vi "ProdaNG.Tree.Selection.GetAll.vi"(7 "TestStepsTree":refnum<vi>, 8 "error in (no error)":errorcluster) -> (0 "error out":errorcluster, 1 "Selected elements values":T1[](array[typedef]), 2 "Selected elements":T2[](array[typedef]))   [LabVIEW 2016]
uses:
  ProdaNG.Tree.Fglb.Data.ctl
  ProdaNG.Tree.Fglb.Element.ctl
  ProdaNG.Tree.Fglb.Value.ctl
  ProdaNG.Tree.Fglb.Action.ctl
  ProdaNG.Configurator.Glb.vi
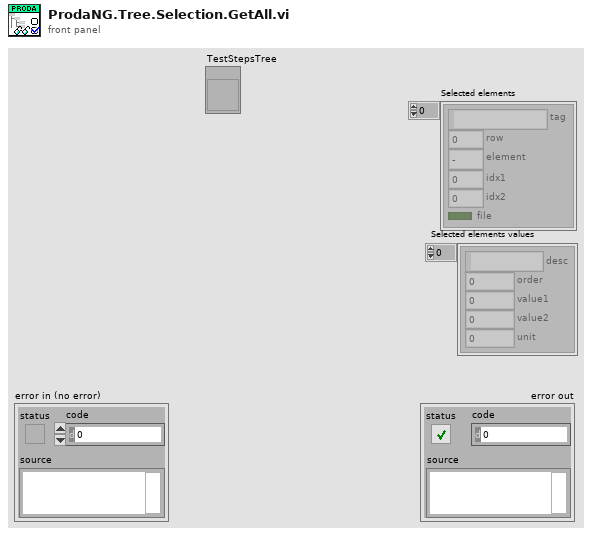
[diagram p1: front panel]
types:
  T1 = typedef "ProdaNG.Tree.Fglb.Value.ctl" = cluster{"desc":string, "order":i32, "value1":dbl, "value2":dbl, "unit":i32}
  T2 = typedef "ProdaNG.Tree.Fglb.Data.ctl" = cluster{"tag":string, "row":i32, "element":T3, "idx1":i32, "idx2":i32, "file":bool}
  T3 = typedef "ProdaNG.Tree.Fglb.Element.ctl" = enum16{"-", "PP", "TS", "TP", "TV"}
  T4 = typedef "ProdaNG.Tree.Fglb.Action.ctl" = enum16{"init", "add", "get by row", "get by tag", "get by idx"}
  T5 = typedef "ProdaNG.ProcessStepParam.ctl" = cluster{"i_id":i32, "processStepId":i32, "unitId":i32, "contentId":string, "previewId":string, "value":dbl, "valueText":string, "paramSequence":i32, "history":i32, "mdReason":string, "mdUser":string, "mdTime":string, "description":string}
  T6 = cluster{"description":string, "paramSequence":i32, "value":dbl, dbl, "unitId":i32}
  T7 = typedef "ProdaNG.TestStep.ctl" = cluster{"i_id":i32, "processStepId":i32, "testSequence":i32, "testOrder":i32, "mdReason":string, "mdUser":string, "mdTime":string, "description":string}
  T8 = typedef "ProdaNG.TestStepParam.ctl" = cluster{"i_id":i32, "testStepId":i32, "unitId":i32, "contentId":string, "previewId":string, "value":dbl, "valueText":string, "paramSequence":i32, "history":i32, "mdReason":string, "mdUser":string, "mdTime":string, "description":string}
  T9 = typedef "ProdaNG.TestValue.ctl" = cluster{"i_id":i32, "testStepId":i32, "releaseId":i32, "unitId":i32, "contentId":string, "previewId":string, "maximum":dbl, "minimum":dbl, "valueText":string, "testValueSequence":i32, "history":i32, "mdReason":string, "mdUser":string, "mdTime":string, "description":string}
  T10 = cluster{"description":string, "testSequence":i32, dbl, dbl, "unitId":i32}
  T11 = cluster{"description":string, "testValueSequence":i32, "minimum":dbl, "maximum":dbl, "unitId":i32}
  T12 = cluster{"element":T3, "found entry":T2, cluster{"description":string, "testValueSequence":i32, "minimum":dbl, "maximum":dbl, "unitId":i32}}
  T13 = cluster{"element":T3, "found entry":T2, cluster{"description":string, "testValueSequence":i32, "minimum":dbl, "maximum":dbl, "unitId":i32}}[]
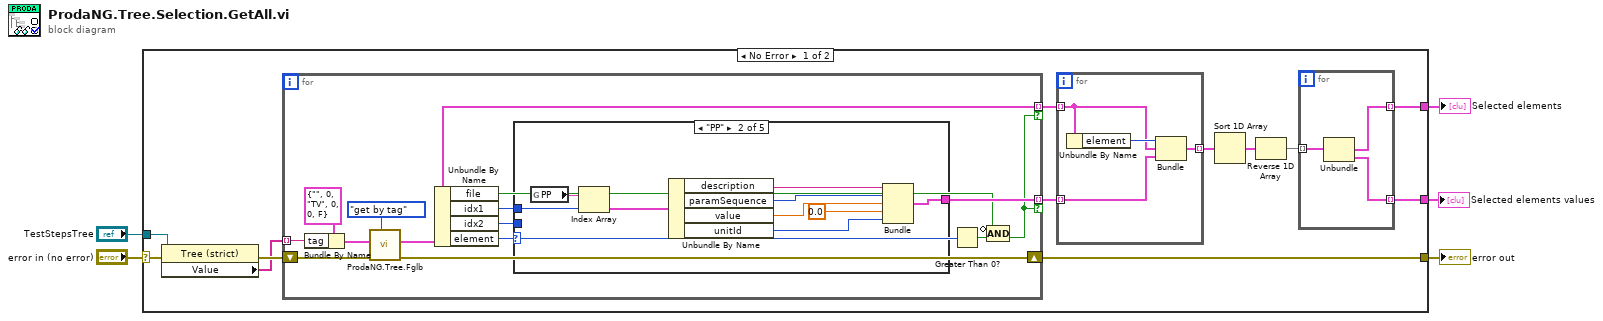
[diagram p0: block diagram]
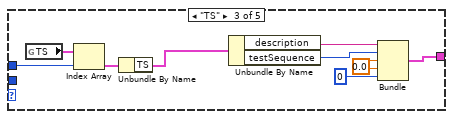
[diagram p3: hidden frame]
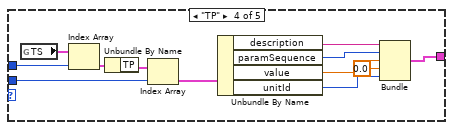
[diagram p4: hidden frame]
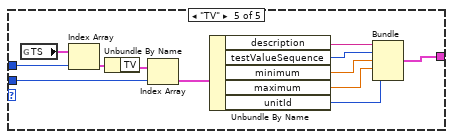
[diagram p5: hidden frame]
diagram:
  n1 = case shown="No Error" "error in (no error)" {
    selector: "error in (no error)" -> [w17 w81]
    tunnel: "TestStepsTree" -> [w14 _]
    tunnel: [w15 w81] -> w5
    tunnel: [w8 _] -> w2
    tunnel: [w6 _] -> w1
    frame No Error {
      n2 = property on="Property Node" class="Tree (strict)"(reference=w14, error in=w17) -> (error out=w16:errorcluster, "Value"=w13:string[])  [unwired: 1 out]
      n3 = for {
        tunnel: w13 -> [w35] mode=indexing
        shift-right: [w32] -> w15
        shift-left: w16 -> [w34]
        tunnel: [w33] -> w9 mode=indexing if=w26
        tunnel: [w29] -> w7 mode=indexing if=w26
        n4 = Bundle By Name(cluster=T2 {"tag"="", "row"=0, "element"=enum."TV", "idx1"=0, "idx2"=0, "file"=FALSE} ("entry in"), "tag"=w35) -> (w36:T2)
        n5 = call "ProdaNG.Tree.Fglb.vi"("Action (add)"=ProdaNG.Tree.Fglb.Action."get by tag", "error in"=w34, "entry in"=w36) -> ("error out"=w32:errorcluster, "found entry"=w33:T2)  [unwired: 6 in, 1 out]
        n6 = Unbundle By Name(w33) -> ("file"=w25:bool, "idx1"=w30:i32, "idx2"=w31:i32, "element"=w28:T3)
        n7 = case shown="\"PP\"" w28 {
          tunnel: w31 -> [_ _ _ w65 w77]
          tunnel: w30 -> [_ w44 w53 w64 w76]
          tunnel: [_ w42 w50 w60 w72] -> w29
          frame "-" {
          }
          frame "PP" {
            n8 = global read "ProdaNG.Configurator.Glb.vi" "PP"() -> (w47:T5[])
            n9 = Index Array(array=w47, index=w44) -> (element=w43:T5)
            n10 = Unbundle By Name(w43) -> ("description"=w46:string, "paramSequence"=w45:i32, "value"=w41:dbl, "unitId"=w39:i32)
            n11 = Bundle("description"=w46, "paramSequence"=w45, "value"=w41, 0.0, "unitId"=w39) -> (w42:T6)  [unwired: 1 in]
          }
          frame "TS" {
            w51 = 0.0
            n12 = global read "ProdaNG.Configurator.Glb.vi" "TS"() -> (w56:cluster{"TS":T7, "TP":T8[], "TV":T9[]}[])
            n13 = Index Array(array=w56, index=w53) -> (element=w52:cluster{"TS":T7, "TP":T8[], "TV":T9[]})
            n14 = Unbundle By Name(w52) -> ("TS"=w49:T7)
            n15 = Unbundle By Name(w49) -> ("description"=w55:string, "testSequence"=w54:i32)
            n16 = Bundle("description"=w55, "testSequence"=w54, w51, w51, "unitId"=0) -> (w50:T10)  [unwired: 1 in]
          }
          frame "TP" {
            n17 = global read "ProdaNG.Configurator.Glb.vi" "TS"() -> (w68:cluster{"TS":T7, "TP":T8[], "TV":T9[]}[])
            n18 = Index Array(array=w68, index=w64) -> (element=w67:cluster{"TS":T7, "TP":T8[], "TV":T9[]})
            n19 = Unbundle By Name(w67) -> ("TP"=w66:T8[])
            n20 = Index Array(array=w66, index=w65) -> (element=w63:T8)
            n21 = Unbundle By Name(w63) -> ("description"=w62:string, "paramSequence"=w61:i32, "value"=w59:dbl, "unitId"=w57:i32)
            n22 = Bundle("description"=w62, "paramSequence"=w61, "value"=w59, 0.0, "unitId"=w57) -> (w60:T6)  [unwired: 1 in]
          }
          frame "TV" {
            n23 = global read "ProdaNG.Configurator.Glb.vi" "TS"() -> (w80:cluster{"TS":T7, "TP":T8[], "TV":T9[]}[])
            n24 = Index Array(array=w80, index=w76) -> (element=w79:cluster{"TS":T7, "TP":T8[], "TV":T9[]})
            n25 = Unbundle By Name(w79) -> ("TV"=w78:T9[])
            n26 = Index Array(array=w78, index=w77) -> (element=w75:T9)
            n27 = Unbundle By Name(w75) -> ("description"=w74:string, "testValueSequence"=w73:i32, "minimum"=w71:dbl, "maximum"=w70:dbl, "unitId"=w69:i32)
            n28 = Bundle("description"=w74, "testValueSequence"=w73, "minimum"=w71, "maximum"=w70, "unitId"=w69) -> (w72:T11)  [unwired: 1 in]
          }
        }
        n29 = Greater Than 0?(x=w28) -> (x > 0?=w27:bool)
        n30 = Compound Arithmetic op=AND(invert w25, w27) -> (w26:bool)
      }
      n31 = for {
        tunnel: w9 -> [w23] mode=indexing
        tunnel: w7 -> [w21] mode=indexing
        tunnel: [w22] -> w12 mode=indexing
        n32 = Unbundle By Name(w23) -> ("element"=w24:T3)
        n33 = Bundle("element"=w24, "found entry"=w23, w21) -> (w22:T12)  [unwired: 1 in]
      }
      n34 = Sort 1D Array(array=w12) -> (sorted array=w11:T13)
      n35 = Reverse 1D Array(array=w11) -> (reversed array=w10:T13)
      n36 = for {
        tunnel: w10 -> [w20] mode=indexing
        tunnel: [w19] -> w8 mode=indexing
        tunnel: [w18] -> w6 mode=indexing
        n37 = Unbundle(w20) -> ("found entry"=w19:T2, w18:T11)  [unwired: 1 out]
      }
    }
    frame Error {
    }
  }
  "error out" <- w5
  "Selected elements" <- w2
  "Selected elements values" <- w1
